vi "Clean LDA -ve Arrival time traces.vi"(3 "LDA Data In":dbl[][](array[numeric])) -> (0 "Negative Arrival Time":bool, 1 "LDA Data Out":dbl[][](array[numeric]))   [LabVIEW 2020]
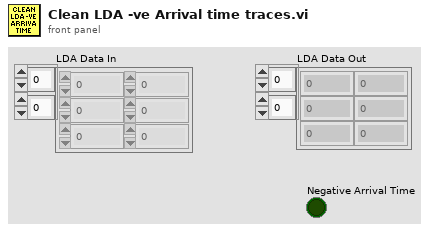
[diagram p1: front panel]
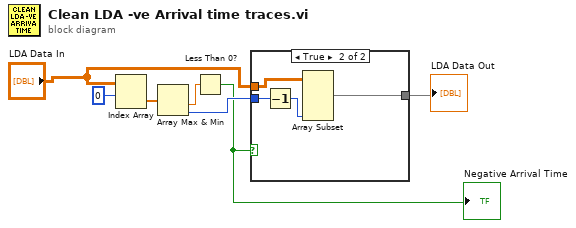
[diagram p0: block diagram]
diagram:
  n1 = Index Array(array="LDA Data In", index (row)=0) -> (element=w4:dbl[])  [unwired: 1 in]
  n2 = Array Max & Min(array=w4) -> (min value=w5:dbl, min index (indices)=w7:i32)  [unwired: 2 out]
  n3 = Less Than 0?(x=w5) -> (x < 0?=w6:bool)
  "Negative Arrival Time" <- w6
  n4 = case shown="True" w6 {
    tunnel: w7 -> [_ w12]
    tunnel: "LDA Data In" -> [w8 w11]
    tunnel: [w8 w9] -> w1
    frame False {
    }
    frame True {
      n5 = Decrement(x=w12) -> (x-1=w10:i32)
      n6 = Array Subset(array=w11, length (col)=w10) -> (w9:dbl[][])  [unwired: 3 in]
    }
  }
  "LDA Data Out" <- w1
